vi "WPI_CameraSend Images To PC Loop - Fix.vi"(8 "error in (no error)":errorcluster, 9 "port":u16=1181, 10 "IP CGI string":string="/axis-cgi/mjpg/video.cgi") -> ()   [LabVIEW 2018]
doc: "This VI is used to serve images from one or more named cameras on your robot to the dashboard, SmartDashboard, or compatible web browser. Camera name and type info is published using network tables. Connections are on port 1181 by default and the URL for streaming can be found by looking at the network \"camera\"/streams variable. Cameras that are opened and stored in the name registry are automatically published by that name.\n\nThis VI runs in parallel with other code and should be placed in Robot Main or in Periodic Tasks.\n\nThis software is licensed. Open the labview\\readme\\WPI Robotics Library Open Source License.txt file for more information."
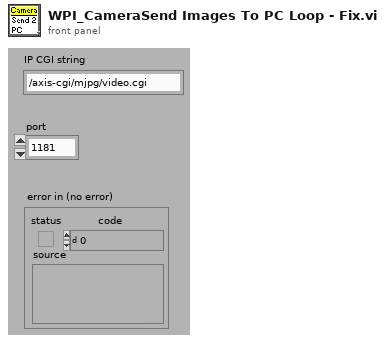
[diagram p1: front panel]
types:
  T1 = enum16{"Standard", "Buffered", "CRLF", "Immediate"}
  T2 = cluster{"token string":string, "token string 2":string}[]
  T3 = cluster{"Type":u32, "Version":u32, "Flags":u32, "SerialNumberHigh":u32, "SerialNumberLow":u32, "BusType":u32, "InterfaceName":string, "VendorName":string, "ModelName":string, "CameraFileName":string, "CameraAttributeURL":string}[]
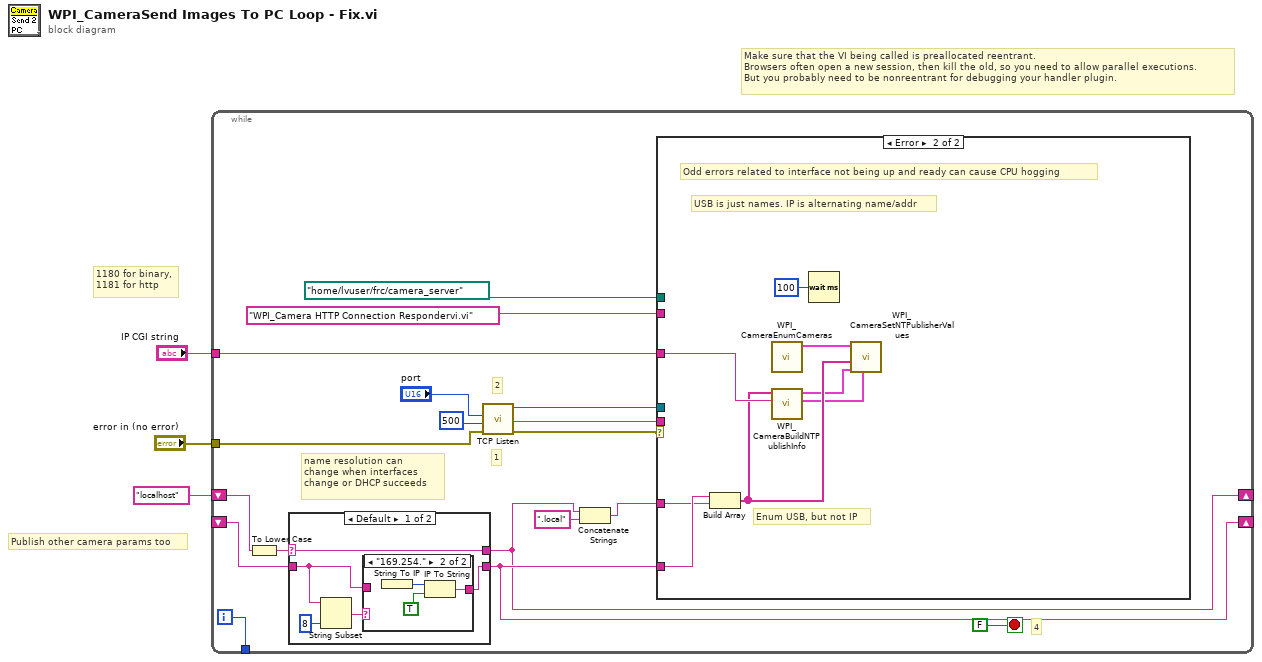
[diagram p0: block diagram]
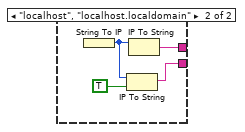
[diagram p3: hidden frame]
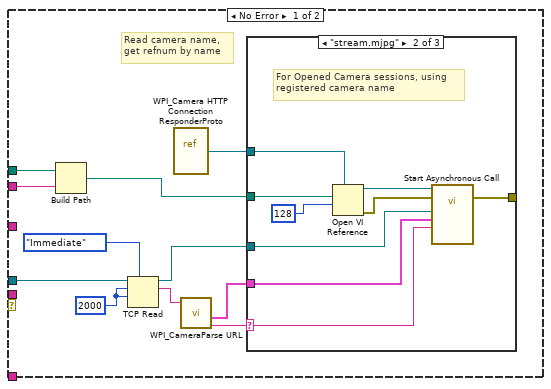
[diagram p4: hidden frame]
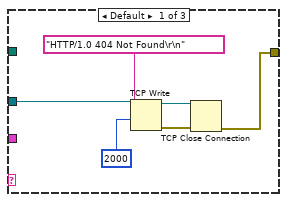
[diagram p5: hidden frame]
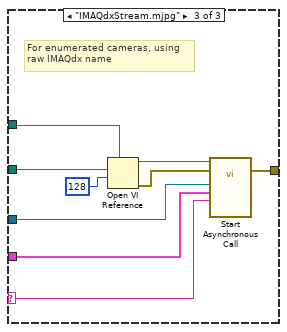
[diagram p6: hidden frame]
diagram:
  # "Make sure that the VI being called is preallocated reentrant.\nBrowsers often open a new session, then kill the old, so you need to allow parallel executions.\nBut you probably need to be nonreentrant for debugging your handler plugin."
  # "Publish other camera params too"
  # "1180 for binary,\n1181 for http"
  n1 = while {
    tunnel: "error in (no error)" -> [w20]
    tunnel: [w15] -> _
    shift-right: [w6] -> _
    shift-left: "localhost" -> [w12]
    shift-right: [w10] -> _
    shift-left: _ -> [w11]
    tunnel: "IP CGI string" -> [w9]
    i -> [w15]
    stop <- FALSE ("status") stop-if-true
    # "name resolution can\nchange when interfaces\nchange or DHCP succeeds"
    # "4"
    # "1"
    # "2"
    n2 = To Lower Case(string=w12) -> (all lower case string=w13:string)
    n3 = case shown="Default" w13 {
      selector: w13 -> [w26 _]
      tunnel: [w26 w34] -> w6
      tunnel: w11 -> [w23 _]
      tunnel: [w22 w31] -> w10
      frame Default {
        n4 = String Subset(string=w23, length (rest)=8 ("length (rest)")) -> (substring=w24:string)  [unwired: 1 in]
        n5 = case shown="\"169.254.\"" w24 {
          tunnel: w23 -> [w27 _]
          tunnel: [w27 w28] -> w22
          frame Default {
          }
          frame "169.254." {
            n6 = String To IP() -> (0:w30:u32)  [unwired: 1 in]
            n7 = IP To String(1:TRUE ("dot notation? (F)"), 2:w30) -> (0:w28:string)
          }
        }
      }
      frame "localhost", "localhost.localdomain" {
        n8 = String To IP() -> (0:w32:u32)  [unwired: 1 in]
        n9 = IP To String(1:TRUE ("dot notation? (F)"), 2:w32) -> (0:w31:string)
        n10 = IP To String(2:w32) -> (0:w34:string)  [unwired: 1 in]
      }
    }
    n11 = call <vilib>:"TCP Listen.vi"("error in (no error)"=w20, "timeout ms (wait forever: -1)"=u16 500 ("port"), "port"="port") -> ("error out"=w17:errorcluster, "remote address"=w21:string, "connection ID"=w19:refnum<k5>)  [unwired: 1 in, 5 out]
    n12 = Concatenate Strings(w6, ".local" ("string")) -> (w5:string)
    n13 = case shown="Error" w17 {
      tunnel: w21 -> [_ _]
      tunnel: w19 -> [w43 _]
      tunnel: w5 -> [_ w75]
      tunnel: w10 -> [_ w76]
      tunnel: w9 -> [_ w74]
      tunnel: "WPI_Camera HTTP Connection Respondervi.vi" -> [w38 _]
      tunnel: path "/home/lvuser/frc/camera_server" -> [w37 _]
      frame No Error {
        w44 = 2000
        # "Read camera name,\nget refnum by name"
        n14 = Build Path(base path=w37, name or relative path=w38) -> (appended path=w36:path)
        n15 = TCP Read(connection ID=w43, bytes to read=w44, 7:T1."Immediate" ("mode (standard)"), 9:w44) -> (connection ID out=w42:refnum<k5>, data out=w40:string)  [unwired: 1 in, 1 out]
        n16 = vi-ref <vilib>:"WPI_Camera HTTP Connection ResponderProto.vi"() -> (w35:refnum<vi>)
        n17 = call <vilib>:"WPI_CameraParse URL.vi"("URL"=w40) -> ("cgi string"=w39:string, "parameters"=w41:T2)  [unwired: 7 in, 2 out]
        n18 = case shown="\"stream.mjpg\"" w39 {
          selector: w39 -> [_ w53 w62]
          tunnel: w36 -> [_ w60 w69]
          tunnel: w42 -> [w51 w58 w67]
          tunnel: [w46 w56 w65] -> _
          tunnel: w41 -> [_ w55 w64]
          tunnel: w35 -> [_ w52 w61]
          frame Default {
            n19 = TCP Write(connection ID=w51, data in="HTTP/1.0 404 Not Found\r\n" ("regular expression"), 9:2000) -> (connection ID out=w50:refnum<k5>, error out=w47:errorcluster)  [unwired: 1 in, 1 out]
            n20 = TCP Close Connection(connection ID=w50, error in (no error)=w47) -> (error out=w46:errorcluster)  [unwired: 2 out]
          }
          frame "stream.mjpg" {
            # "For Opened Camera sessions, using\nregistered camera name"
            n21 = Open VI Reference(type specifier VI Refnum (for type only)=w52, vi path=w60, options=128) -> (vi reference=w54:refnum<vi>, error out=w57:errorcluster)  [unwired: 3 in]
            n22 = call-by-ref "Start Asynchronous Call"(reference=w54, error in=w57, "CGI String"=w53, "parameters"=w55, "connection ID"=w58) -> (error out=w56:errorcluster)  [unwired: 9 in, 1 out]
          }
          frame "IMAQdxStream.mjpg" {
            # "For enumerated cameras, using\nraw IMAQdx name"
            n23 = Open VI Reference(type specifier VI Refnum (for type only)=w61, vi path=w69, options=128) -> (vi reference=w63:refnum<vi>, error out=w66:errorcluster)  [unwired: 3 in]
            n24 = call-by-ref "Start Asynchronous Call"(reference=w63, error in=w66, "CGI String"=w62, "parameters"=w64, "connection ID"=w67) -> (error out=w65:errorcluster)  [unwired: 9 in, 1 out]
          }
        }
      }
      frame Error {
        # "Enum USB, but not IP"
        # "USB is just names. IP is alternating name/addr"
        # "Odd errors related to interface not being up and ready can cause CPU hogging"
        n25 = Build Array(w76, w75) -> (w72:string[])
        n26 = call <vilib>:"WPI_CameraEnumCameras.vi"() -> ("USB Cams"=w73:T3)  [unwired: 10 in, 1 out]
        n27 = call <vilib>:"WPI_CameraBuildNTPublishInfo.vi"("IP CGI string"=w74, "RIO Addresses"=w72) -> ("Streams"=w70:cluster{string, "URLs":string[]}[], "Sources"=w71:cluster{string, string}[])  [unwired: 8 in]
        n28 = Wait (ms)(milliseconds to wait=u32 100) -> ()  [unwired: 1 out]
        n29 = call <vilib>:"WPI_CameraSetNTPublisherValues.vi"("Streams"=w70, "Sources"=w71, "roboRIO Addresses"=w72, "USB Cams"=w73) -> ()  [unwired: 8 in]
      }
    }
  }
